vi "GetAppRefInCluster.vi"() -> (0 "error out":errorcluster, 1 "Cluster":cluster{"App Refnum":refnum<vi>})   [LabVIEW 2012]
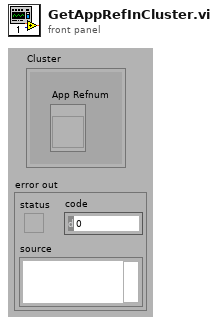
[diagram p1: front panel]
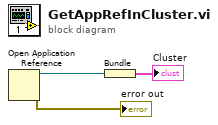
[diagram p0: block diagram]
diagram:
  n1 = Open Application Reference() -> (0:→"error out":errorcluster, 3:w2:refnum<vi>)  [unwired: 1 in, 3 out]
  n2 = Bundle("application reference"=w2) -> (→"Cluster":cluster{"application reference":refnum<vi>})  [unwired: 1 in]
